vi "EnviarDatosFireBase.vi"() -> ()   [LabVIEW 2025]
uses:
  <vilib>/httpClient/PUTBuffer.vi
  <vilib>/httpClient/LabVIEWHTTPClient.lvlib
panel:
  in  "stop":bool
  out "error out":errorcluster
  out "body":string
  out "headers":string
  in  "rele":bool
  in  "accionamiento":dbl(knob) scale=0.0..10.0
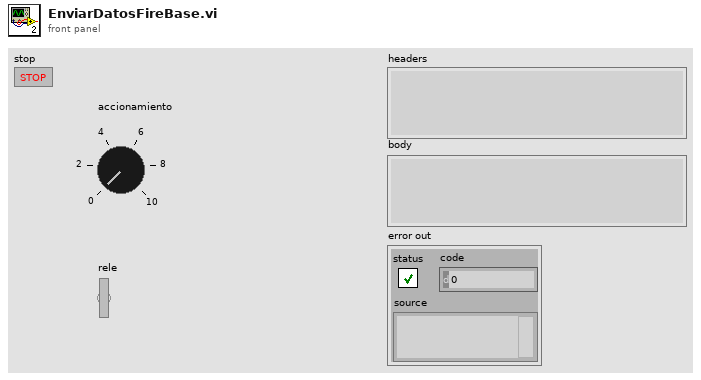
[diagram p1: front panel]
types:
  T1 = cluster{"accionamiento":dbl, "fecha":string, "hora":string, "rele":bool}
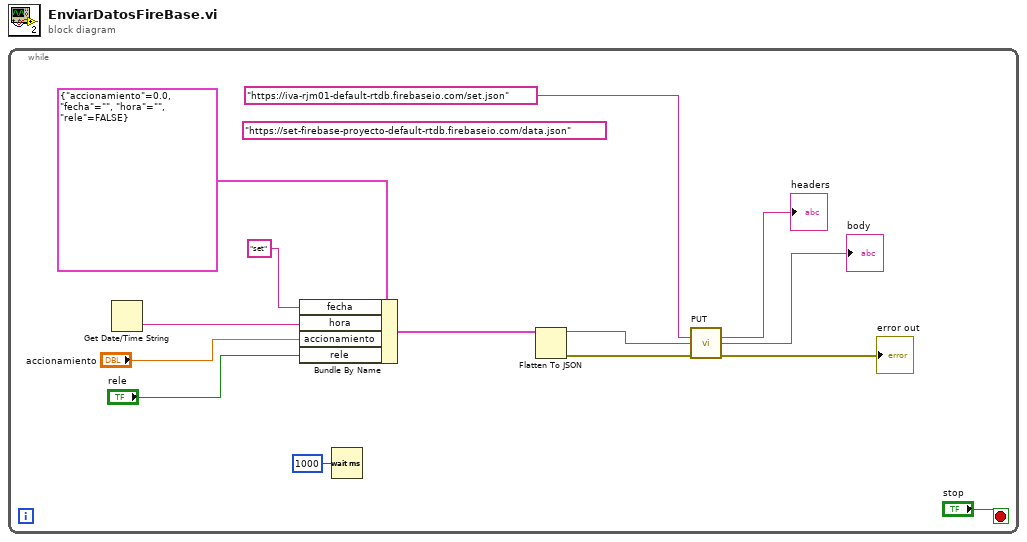
[diagram p0: block diagram]
diagram:
  n1 = while {
    stop <- "stop" stop-if-true
    (unwired) "https://set-firebase-proyecto-default-rtdb.firebaseio.com/data.json"
    n2 = Get Date/Time String() -> (time string=w14:string)  [unwired: 3 in, 1 out]
    n3 = Bundle By Name "Bundle By Name"(cluster=T1 {"accionamiento"=0.0, "fecha"="", "hora"="", "rele"=FALSE}, "fecha"="set", "hora"=w14, "accionamiento"="accionamiento", "rele"="rele") -> (w9:T1)
    n4 = Wait (ms)(milliseconds to wait=u32 1000) -> ()  [unwired: 1 out]
    n5 = Flatten To JSON(anything=w9) -> (JSON string=w7:string, 11:w8:errorcluster)  [unwired: 2 in]
    n6 = call-poly <vilib>:"PUT.vi"("url"="https://iva-rjm01-default-rtdb.firebaseio.com/set.json", "buffer"=w7, "error in (no error)"=w8) -> ("headers"=→"headers":string, "body"=→"body":string, "error out"=→"error out":errorcluster)  [unwired: 9 in, 1 out]
  }
